vi "callback_recv.vi"(8 "error in (no error)":errorcluster, 9 "flags":i32, 10 "length":u64, 11 "socket":u64) -> (0 "error out":errorcluster, 1 "buffer":u8[](array[numeric]), 2 "bytes received":i64)   [LabVIEW 2013, in "libssh2_integration_tests.lvlib"]
doc: "Called when libssh2 wants to read data from the connection.\n\n<B>socket</B> the socket to read from.\n<B>length</B> number of bytes to read from the connection.\n<B>flags</B> flags that would have been used by a send() call.\n\nReturns the actual number of bytes received and the received bytes."
uses:
  libssh2_integration_tests.lvlib
  ws2_32.dll
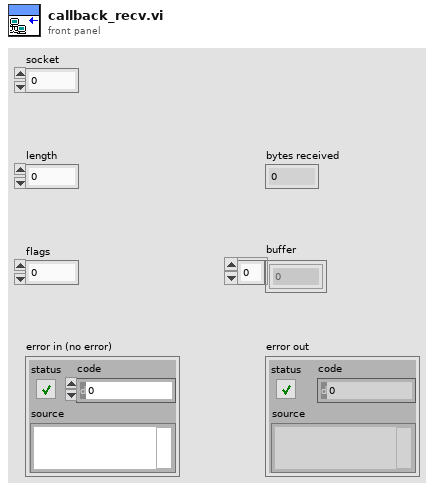
[diagram p1: front panel]
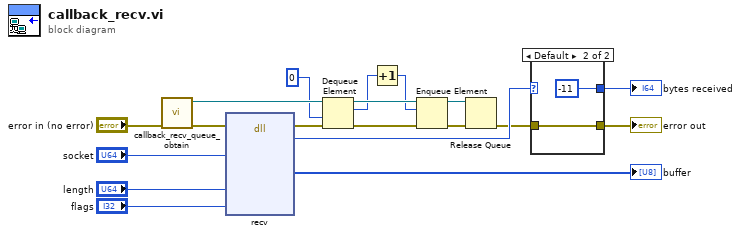
[diagram p0: block diagram]
diagram:
  n1 = call "callback_recv_queue_obtain.vi"("error in (no error)"="error in (no error)") -> ("error out"=w12:errorcluster, "queue out"=w10:refnum<queue>)  [unwired: 9 in]
  n2 = dll-call lib="ws2_32.dll" fn="recv"(error in=w12, "s"="socket", "len"="length", "flags"="flags") -> (error out=w14:errorcluster, "return type"=w9:i32, "buf"=→"buffer":u8[])  [unwired: 6 in, 1 out]
  n3 = Dequeue Element(queue=w10, timeout in ms (-1)=0, error in (no error)=w14) -> (queue out=w5:refnum<queue>, element=w4:i32, error out=w11:errorcluster)  [unwired: 1 out]
  n4 = Increment(x=w4) -> (x+1=w3:i32)
  n5 = Enqueue Element(queue=w5, element=w3, error in (no error)=w11) -> (queue out=w6:refnum<queue>, error out=w7:errorcluster)  [unwired: 1 in, 1 out]
  n6 = Release Queue(queue=w6, error in (no error)=w7) -> (error out=w8:errorcluster)  [unwired: 1 in, 2 out]
  n7 = case shown="Default" w9 {
    selector: w9 -> [w21 _]
    tunnel: w8 -> [w20 w23]
    tunnel: [w20 w23] -> w13
    tunnel: [w21 -11] -> w1
    frame 0.. {
    }
    frame Default {
    }
  }
  "error out" <- w13
  "bytes received" <- w1
